vi "Logic Check.vi"(0 "STEP in":T1, 1 "Variables State in":T10, 2 "HW InOut MAP":T11, 3 "STEP State in":T9, 4 "Notifiers.Control":T12, 5 "error in (no error)":errorcluster, 6 "Current Sequence":T7) -> (14 "STEP Out":T1, 15 "Variables State out":T10, 16 "HW CTRL Data":T6, 17 "Alarms triggered?":T8, 18 "STEP State out":T9, 19 "error out":errorcluster)   [LabVIEW 2014, in "SeqLoop.lvlib"]
doc: "Mapea las entradas digitales. Chequea el estado de las Variables. Resuelve las operaciones lógicas involucradas en el paso. Detecta Errores y Alarmas, primarias y secundarias. Gestiona el estado del Paso."
uses:
  APIs/Data Queue/Control Data Cluster.ctl
  TypeDefs/HW Variables State.ctl
  TypeDefs/HW InOut MAP.ctl
  TypeDefs/STEP State.ctl
  TypeDefs/Sequence.ctl
  TypeDefs/STEP.ctl
  TypeDefs/LogicParsedExpression.ctl
  Mimico Display/TypeDefs/Mimic Data.ctl
  Mimico Display/TypeDefs/BG Image.ctl
  Mimico Display/TypeDefs/mObject.ctl
  TypeDefs/HW CTRL Data.ctl
  SeqLoop.lvlib
  APIs/Data Queue/WINFAS 2 Data Queue.lvlib
  Mimico Display/Mimico Display.lvlib
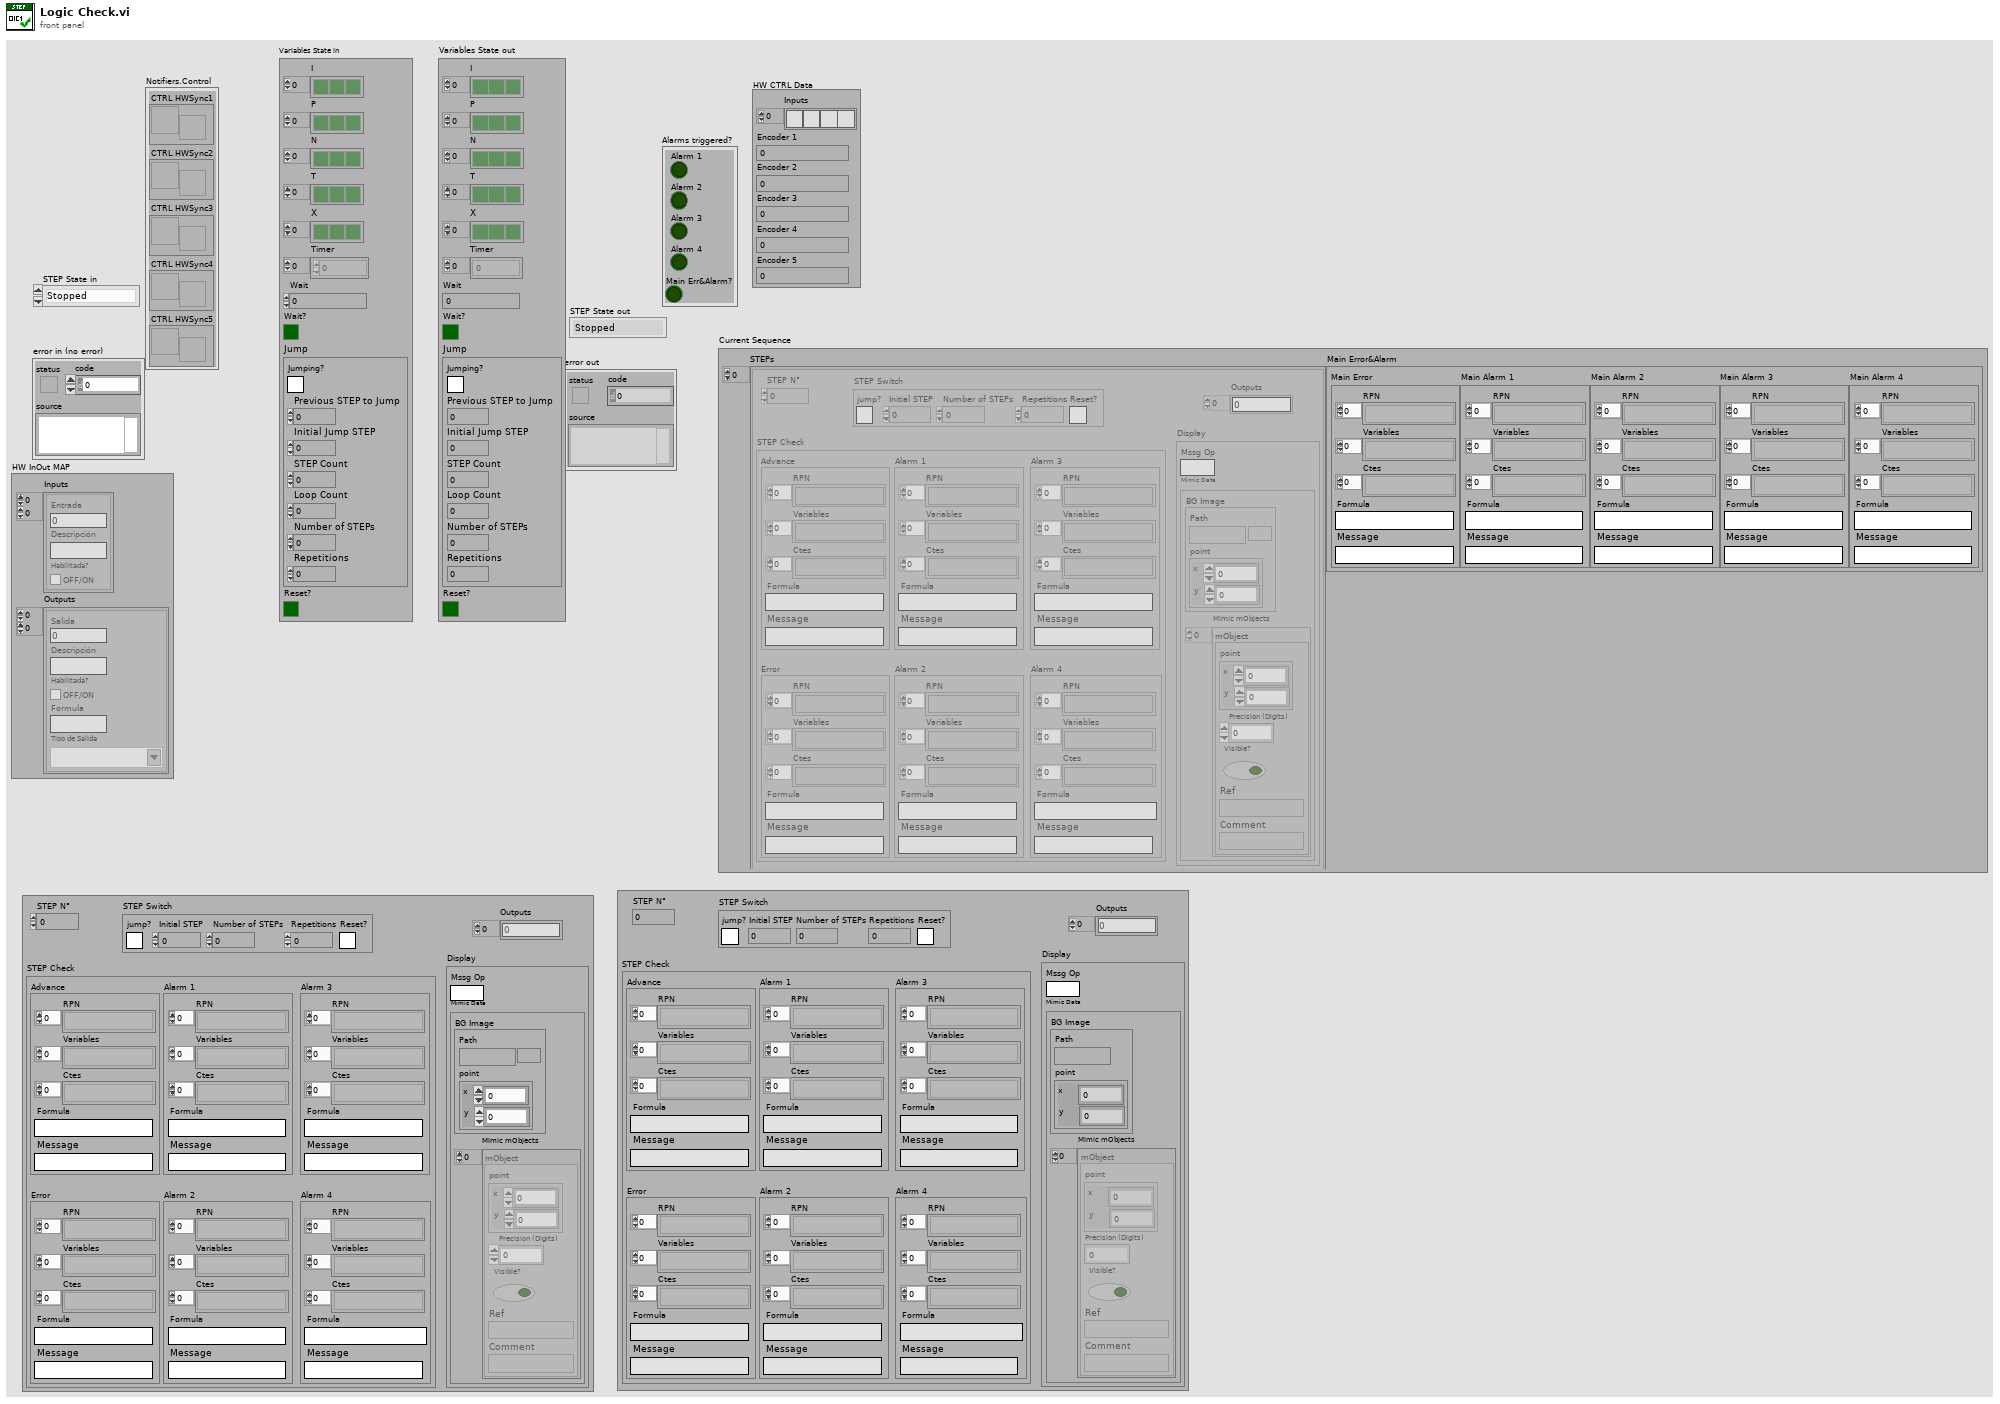
[diagram p1: front panel]
types:
  T1 = typedef "SeqLoop.lvlib/STEP.ctl" = cluster{"STEP N°":u32, "STEP Switch":cluster{"jump?":bool, "Initial STEP":u32, "Number of STEPs":u32, "Repetitions":u32, "Reset?":bool}, "Outputs":i32[], "STEP Check":cluster{"Advance":T2, "Error ":T2, "Alarm 1":T2, "Alarm 2":T2, "Alarm 3":T2, "Alarm 4":T2}, "Display":cluster{"Mssg Op":string, "Mimic Data":T3}}
  T2 = typedef "SeqLoop.lvlib/LogicParsedExpression.ctl" = cluster{"RPN ":string[], "Variables":string[], "Ctes":string[], "Formula":string, "Message":string}
  T3 = typedef "SeqLoop.lvlib/Mimico Display.lvlib/Mimic Data.ctl" = cluster{"BG Image":T4, "Mimic mObjects":T5[]}
  T4 = typedef "SeqLoop.lvlib/Mimico Display.lvlib/BG Image.ctl" = cluster{"Path":path, "point":cluster{"x":i16, "y":i16}}
  T5 = typedef "SeqLoop.lvlib/Mimico Display.lvlib/mObject.ctl" = cluster{"point":cluster{"x":i16, "y":i16}, "Precision (Digits)":i32, "Visible?":bool, "Ref":string, "Comment":string}
  T6 = typedef "SeqLoop.lvlib/HW CTRL Data.ctl" = cluster{"Inputs":bool[], "Encoder 1":sgl, "Encoder 2":sgl, "Encoder 3":sgl, "Encoder 4":sgl, "Encoder 5":sgl}
  T7 = typedef "SeqLoop.lvlib/Sequence.ctl" = cluster{"STEPs":T1[], "Main Error&Alarm":cluster{"Main Error":T2, "Main Alarm 1":T2, "Main Alarm 2":T2, "Main Alarm 3":T2, "Main Alarm 4":T2}}
  T8 = cluster{"Alarm 1":bool, "Alarm 2":bool, "Alarm 3":bool, "Alarm 4":bool, "Main Err&Alarm?":bool}
  T9 = typedef "SeqLoop.lvlib/STEP State.ctl" = enum16{"Stopped", "First Call", "Idle...", "Advance OK", "Alarm", "Output Security", "Error"}
  T10 = typedef "SeqLoop.lvlib/HW Variables State.ctl" = cluster{"I":bool[], "P":bool[], "N":bool[], "T":bool[], "X":bool[], "Timer":u32[], "Wait":u32, "Wait?":bool, "Jump":cluster{"Jumping?":bool, "Previous STEP to Jump":u32, "Initial Jump STEP":u32, "STEP Count":u32, "Loop Count":u32, "Number of STEPs":u32, "Repetitions":u32}, "Reset?":bool}
  T11 = typedef "SeqLoop.lvlib/HW InOut MAP.ctl" = cluster{"Inputs":cluster{"Entrada":i32, "Descripción":string, "Habilitada?":bool}[][], "Outputs":cluster{"Salida":i32, "Descripción":string, "Habilitada?":bool, "Formula":string, "Tipo de Salida":string}[][]}
  T12 = cluster{"CTRL HWSync1":refnum<notifier>, "CTRL HWSync2":refnum<notifier>, "CTRL HWSync3":refnum<notifier>, "CTRL HWSync4":refnum<notifier>, "CTRL HWSync5":refnum<notifier>}
  T13 = cluster{"Alarm 1":bool, "Alarm 2":bool, "Alarm 3":bool, "Alarm 4":bool, "Main Alarm?":bool}
  T14 = cluster{"Advance":T2, "Error ":T2, "Alarm 1":T2, "Alarm 2":T2, "Alarm 3":T2, "Alarm 4":T2}
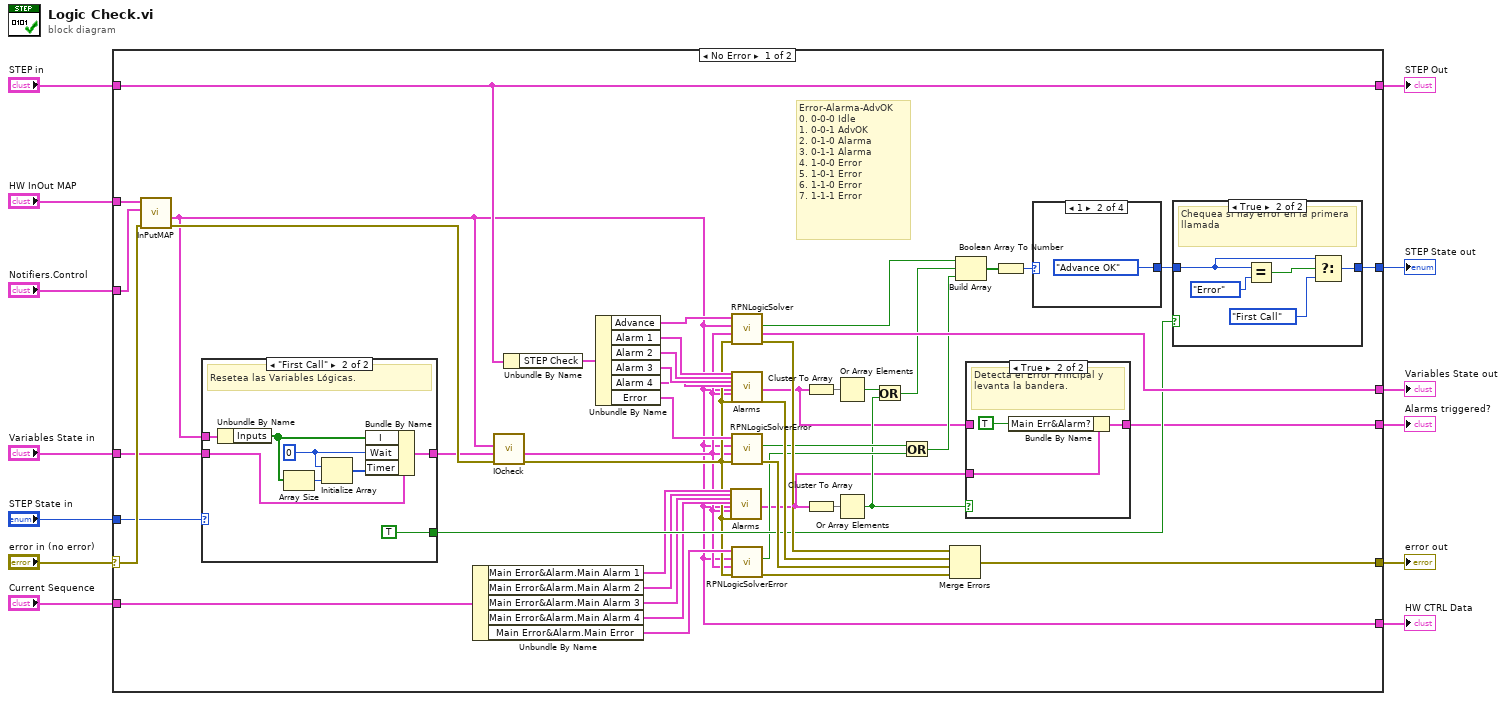
[diagram p0: block diagram]
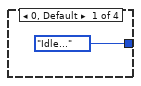
[diagram p4: hidden frame]
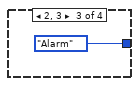
[diagram p5: hidden frame]
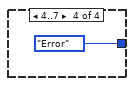
[diagram p6: hidden frame]
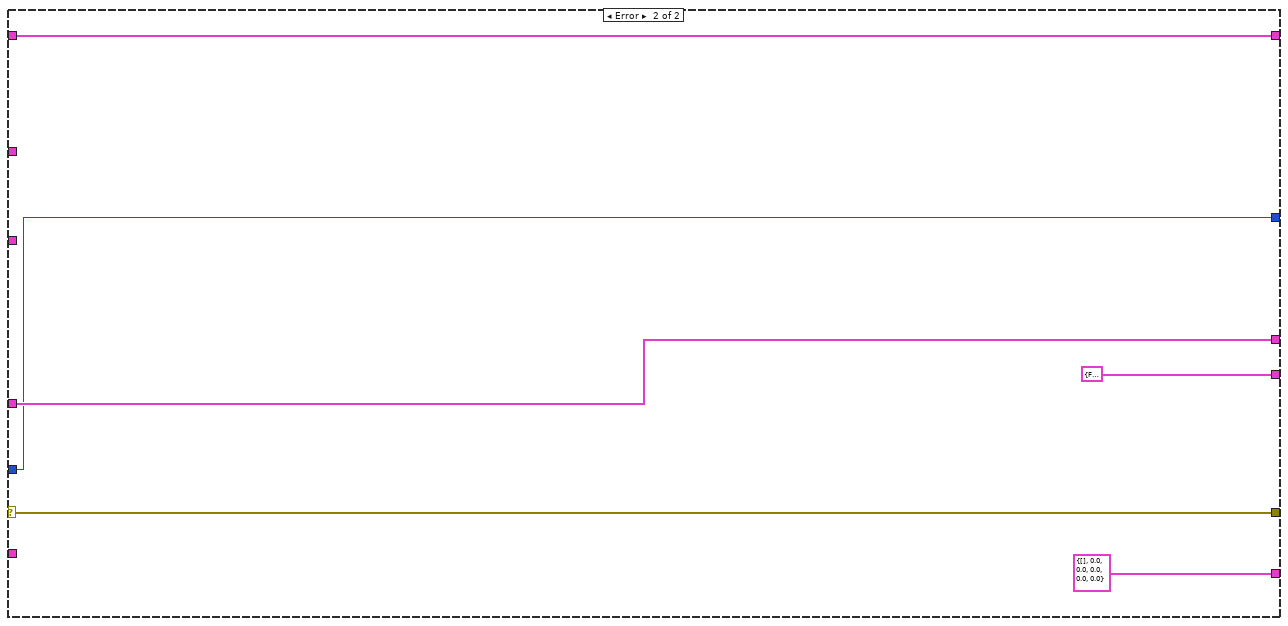
[diagram p8: hidden frame]
diagram:
  n1 = case shown="No Error" "error in (no error)" {
    selector: "error in (no error)" -> [w59 w89]
    tunnel: [w57 w89] -> w12
    tunnel: [w46 w88] -> w1
    tunnel: "STEP in" -> [w46 w88]
    tunnel: "Notifiers.Control" -> [w56 _]
    tunnel: "Variables State in" -> [w55 w87]
    tunnel: "HW InOut MAP" -> [w15 _]
    tunnel: [w42 w87] -> w8
    tunnel: "STEP State in" -> [w38 w86]
    tunnel: [w35 w86] -> w6
    tunnel: "Current Sequence" -> [w34 _]
    tunnel: [w18 T13 {"Alarm 1"=FALSE, "Alarm 2"=FALSE, "Alarm 3"=FALSE, "Alarm 4"=FALSE, "Main Alarm?"=FALSE} ("Alarms triggered?")] -> w4
    tunnel: [w14 T6 {"Inputs"=[], "Encoder 1"=0.0, "Encoder 2"=0.0, "Encoder 3"=0.0, "Encoder 4"=0.0, "Encoder 5"=0.0} ("HW CTRL Data")] -> w3
    frame No Error {
      # "Error-Alarma-AdvOK\n0. 0-0-0 Idle\n1. 0-0-1 AdvOK\n2. 0-1-0 Alarma\n3. 0-1-1 Alarma\n4. 1-0-0 Error\n5. 1-0-1 Error\n6. 1-1-0 Error\n7. 1-1-1 Error"
      n2 = call "InPutMAP.vi"("error in (no error)"=w59, "Notifiers.Control"=w56, "Mapping Buss In"=w15) -> ("error out"=w60:errorcluster, "HW CTRL Data"=w14:T6)  [unwired: 7 in]
      n3 = case shown="\"First Call\"" w38 {
        tunnel: [w75 w81] -> w47
        tunnel: w55 -> [w75 w79]
        tunnel: w14 -> [_ w78]
        tunnel: [_ TRUE] -> w37
        frame Default {
        }
        frame "First Call" {
          w82 = u32 0 ("element")
          # "Resetea las Variables Lógicas."
          n4 = Unbundle By Name(w78) -> ("Inputs"=w77:bool[])
          n5 = Array Size(array=w77) -> (size(s)=w80:i32)
          n6 = Initialize Array(w82, w80) -> (w83:u32[])
          n7 = Bundle By Name(cluster=w79, "I"=w77, "Wait"=w82, "Timer"=w83) -> (w81:T10)
        }
      }
      n8 = Unbundle By Name(w34) -> ("Main Error&Alarm.Main Alarm 1"=w29:T2, "Main Error&Alarm.Main Alarm 2"=w28:T2, "Main Error&Alarm.Main Alarm 3"=w27:T2, "Main Error&Alarm.Main Alarm 4"=w26:T2, "Main Error&Alarm.Main Error"=w32:T2)
      n9 = call "IOcheck.vi"("error in (no error)"=w60, "Variables State in"=w47, "HW CTRL Data"=w14) -> ("error out"=w17:errorcluster, "Variables State out"=w16:T10)  [unwired: 7 in]
      n10 = Unbundle By Name(w46) -> ("STEP Check"=w54:T14)
      n11 = Unbundle By Name(w54) -> ("Advance"=w39:T2, "Alarm 1"=w53:T2, "Alarm 2"=w52:T2, "Alarm 3"=w51:T2, "Alarm 4"=w50:T2, "Error"=w44:T2)
      n12 = call "Alarms.vi"("Alarm 1"=w29, "Alarm 2"=w28, "Alarm 3"=w27, "Alarm 4"=w26, "HW CTRL Data"=w14, "Variables State"=w16, "error in (no error)"=w17) -> ("Alarms triggered?"=w19:T8)  [unwired: 19 in, 1 out]
      n13 = call "RPNLogicSolver.vi"("error in"=w17, "Variables State in"=w16, "HW CTRL Data"=w14, "Logic Parsed Expression"=w39) -> ("error out"=w40:errorcluster, "Variables State out"=w42:T10, "Logic Result"=w41:bool)  [unwired: 5 in]
      n14 = call "Alarms.vi"("Alarm 1"=w53, "Alarm 2"=w52, "Alarm 3"=w51, "Alarm 4"=w50, "HW CTRL Data"=w14, "Variables State"=w16, "error in (no error)"=w17) -> ("Alarms triggered?"=w20:T8, "error out"=w58:errorcluster)  [unwired: 19 in]
      n15 = call "RPNLogicSolverError.vi"("error in"=w17, "Variables State in"=w16, "HW CTRL Data"=w14, "Logic Parsed Expression"=w44) -> ("error out"=w43:errorcluster, "Logic Result"=w31:bool)  [unwired: 5 in, 1 out]
      n16 = call "RPNLogicSolverError.vi"("error in"=w17, "Variables State in"=w16, "HW CTRL Data"=w14, "Logic Parsed Expression"=w32) -> ("error out"=w33:errorcluster, "Logic Result"=w30:bool)  [unwired: 5 in, 1 out]
      n17 = Cluster To Array(cluster=w20) -> (array=w45:bool[])
      n18 = Cluster To Array(cluster=w19) -> (array=w25:bool[])
      n19 = Or Array Elements(Boolean array=w45) -> (logical OR=w23:bool)
      n20 = Or Array Elements(Boolean array=w25) -> (logical OR=w21:bool)
      n21 = Or(x=w23, y=w21) -> (x .or. y?=w22:bool)
      n22 = Or(x=w31, y=w30) -> (x .or. y?=w24:bool)
      n23 = Merge Errors(w40, w58, w43, w33) -> (w57:errorcluster)
      n24 = Build Array(w41, w22, w24) -> (w49:bool[])
      n25 = case shown="True" w21 {
        tunnel: w20 -> [w61 _]
        tunnel: w19 -> [_ w64]
        tunnel: [w61 w63] -> w18
        frame False {
        }
        frame True {
          # "Detecta el Error Principal y levanta la bandera."
          n26 = Bundle By Name(cluster=w64, "Main Err&Alarm?"=TRUE) -> (w63:T8)
        }
      }
      n27 = Boolean Array To Number(Boolean array=w49) -> (number=w48:u32)
      n28 = case shown="1" w48 {
        tunnel: [STEP_State."Idle..." ("STEP State out") STEP_State."Advance OK" ("STEP State out") STEP_State."Alarm" ("STEP State out") STEP_State."Error" ("STEP State out")] -> w36
        frame 0, Default {
        }
        frame 1 {
        }
        frame 2, 3 {
        }
        frame 4..7 {
        }
      }
      n29 = case shown="True" w37 {
        tunnel: w36 -> [w65 w68]
        tunnel: [w65 w69] -> w35
        frame False {
        }
        frame True {
          # "Chequea si hay error en la primera llamada"
          n30 = Equal?(x=w68, y=STEP_State."Error") -> (x = y?=w67:bool)
          n31 = Select(t=w68, s=w67, f=STEP_State."First Call") -> (s? t:f=w69:T9)
        }
      }
    }
    frame Error {
    }
  }
  "error out" <- w12
  "Variables State out" <- w8
  "STEP State out" <- w6
  "Alarms triggered?" <- w4
  "HW CTRL Data" <- w3
  "STEP Out" <- w1
